vi "Test Buzzers.vi"(8 "error in (no error)":errorcluster, 10 "Test Mode?":bool, 11 "Controller in":refnum<class "Controller.lvclass">) -> (0 "error out":errorcluster, 3 "Controller out":refnum<class "Controller.lvclass">)   [LabVIEW 2024, in "Controller.lvlib" / "Controller.lvclass"]
uses:
  Controller.lvclass
  C:/Program Files/National Instruments/LabVIEW 2024/vi.lib/ActorFramework/Actor/Actor.lvclass
  Controller.lvclass/Controller.ctl
  <vilib>/ActorFramework/Actor/Actor.lvclass/Actor.ctl
  <vilib>/ActorFramework/Message Enqueuer/Message Enqueuer.lvclass/Message Enqueuer.ctl
  Controller Messages/Question Prompt Display Msg/Question Prompt Display Msg.lvclass/Question Prompt Display Msg.ctl
  <vilib>/ActorFramework/Message Enqueuer/Init from Existing Queue.vi
  <vilib>/ActorFramework/Message Enqueuer/Enqueue.vi
  Controller Messages/Question Prompt Display Msg/Question Prompt Display Msg.lvclass
  C:/Program Files/National Instruments/LabVIEW 2024/vi.lib/ActorFramework/Message/Message.lvclass
  Controller Messages/Load Main Panel Display Msg/Load Main Panel Display Msg.lvclass
  Controller Messages/Reset Contestant Lights Msg/Reset Contestant Lights Msg.lvclass
  <vilib>/ActorFramework/Message Priority Queue/Priority Enqueue.vi
  <vilib>/ActorFramework/Message Enqueuer/Message Enqueuer.lvclass
  <vilib>/ActorFramework/Actor/Actor.lvclass
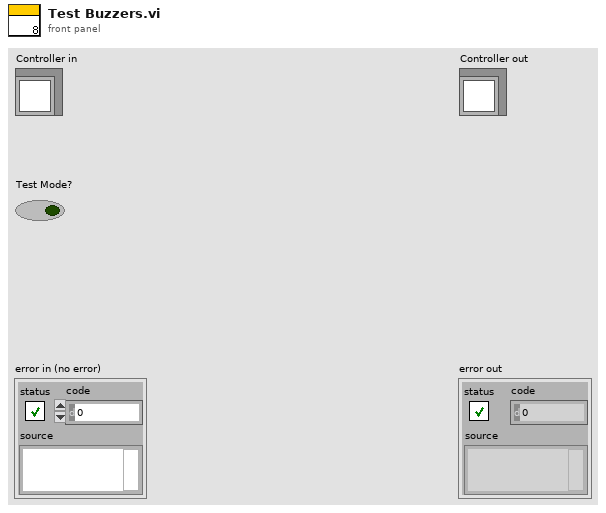
[diagram p1: front panel]
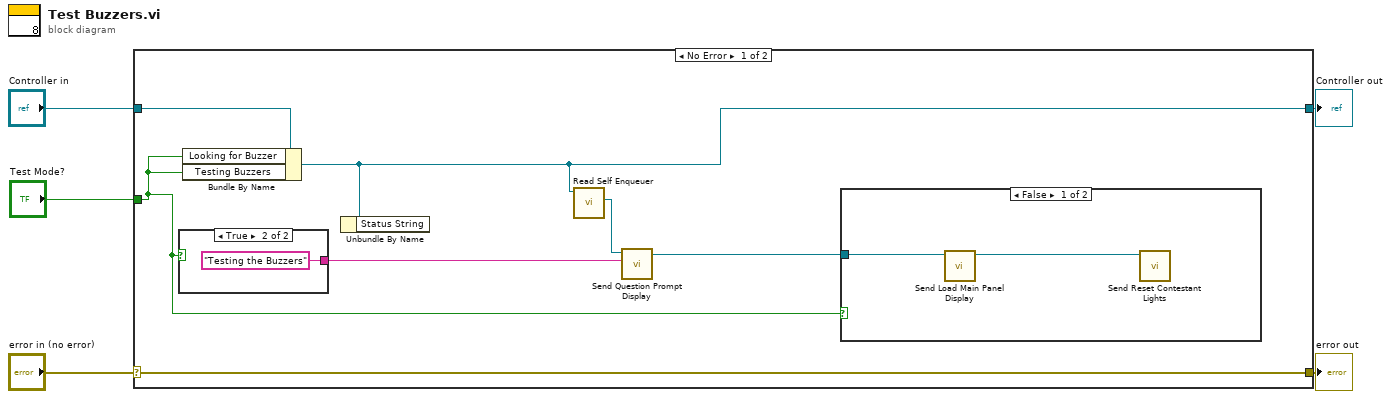
[diagram p0: block diagram]
diagram:
  n1 = case shown="No Error" "error in (no error)" {
    selector: "error in (no error)" -> [w12 w17]
    tunnel: [w12 w17] -> w4
    tunnel: [w10 w16] -> w2
    tunnel: "Controller in" -> [w11 w16]
    tunnel: "Test Mode?" -> [w6 _]
    frame No Error {
      n2 = case shown="True" w6 {
        tunnel: [_ "Testing the Buzzers" ("Value")] -> w8
        frame False {
        }
        frame True {
        }
      }
      n3 = Bundle By Name(cluster=w11, "Looking for Buzzer"=w6, "Testing Buzzers"=w6) -> (w10:refnum<class "Controller.lvclass">)
      n4 = Unbundle By Name(w10) -> ()  [unwired: 1 out]
      n5 = call <vilib>:"Read Self Enqueuer.vi"("Actor"=w10) -> ("Self Enqueuer"=w9:refnum<class "Message Enqueuer.lvclass">)  [unwired: 10 in]
      n6 = call "Send Question Prompt Display.vi"("Prompt"=w8, "Message Enqueuer"=w9) -> ("Message Enqueuer out"=w7:refnum<class "Message Enqueuer.lvclass">)  [unwired: 8 in, 1 out]
      n7 = case shown="False" w6 {
        tunnel: w7 -> [w13 _]
        frame False {
          n8 = call "Send Load Main Panel Display.vi"("Message Enqueuer"=w13) -> ("Message Enqueuer out"=w14:refnum<class "Message Enqueuer.lvclass">)  [unwired: 9 in, 1 out]
          n9 = call "Send Reset Contestant Lights.vi"("Message Enqueuer"=w14) -> ()  [unwired: 9 in, 2 out]
        }
        frame True {
        }
      }
    }
    frame Error {
    }
  }
  "error out" <- w4
  "Controller out" <- w2
